vi "2D Linear Evaluation.vi"(2 "b":dbl format="%0.2f", 3 "a":dbl format="%0.2f", 4 "X":dbl[][](array[numeric]) format="%0.2f") -> (0 "error":i32, 1 "Y=X*a+b":dbl[][](array[numeric]) format="%0.2f")   [LabVIEW 2017, in "NI_AALBase.lvlib"]
doc: "LabVIEW no longer supports this VI. Use the Linear Evaluation VI instead.\nThis VI performs a linear evaluation on the input matrix <b>X</b> using the inputs <b>a</b> and <b>b</b>.\nThis VI calculates <b>Y=X*a+b</b> using the following equation:\nY = <b>aX</b> +<b> b</b>\nwhere <b>a</b> denotes the multiplicative constant and <b>b</b> denotes the additive constant.\nThe following equation defines each element of Y:\nY[i,j] = X[i,j]*a + b."
uses:
  NI_AALBase.lvlib
  <resource>/lvanlys.dll
panel:
  # "Y[i,j]=X[i,j]a+b"
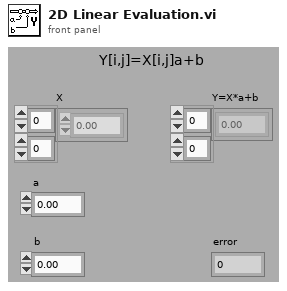
[diagram p1: front panel]
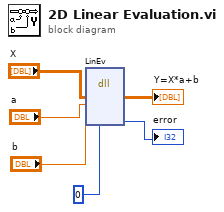
[diagram p0: block diagram]
diagram:
  n1 = dll-call lib="C:/Program Files (x86)/National Instruments/LabVIEW 2017/resource/lvanlys.*" fn="LinEv"("X"="X", "a"="a", "b"="b", 0) -> ("X"=→"Y=X*a+b":dbl[][], →"error":i32)  [unwired: 6 in, 2 out]
